vi "test.vi"() -> ()   [LabVIEW 2014]
panel:
  out "GetDisPlayData":i32(ring) items=["Success", "TimeOut", "CRCError", "WriteOutRange", "DeviceNotOpen", "ExceptionError"]
  out "arrayfloat":sgl[](array[numeric])
  in  "modeCode":i32(ring)=3 items=["CCH"=0, "CCL"=1, "CVH"=2, "CVL"=3, "CR"=4, "CP"=5, "CCDH"=6, "CCDL"=7, "OCP"=8, "DISCHARGE"=9, "AUTO"=12, "SEQ"=13, "LED"=14]
  out "错误输出":errorcluster
  out "Close":bool
  out "Open":bool
  in  "簇":T1
  in  "错误输入（无错误）":errorcluster
  # "-1861025792"
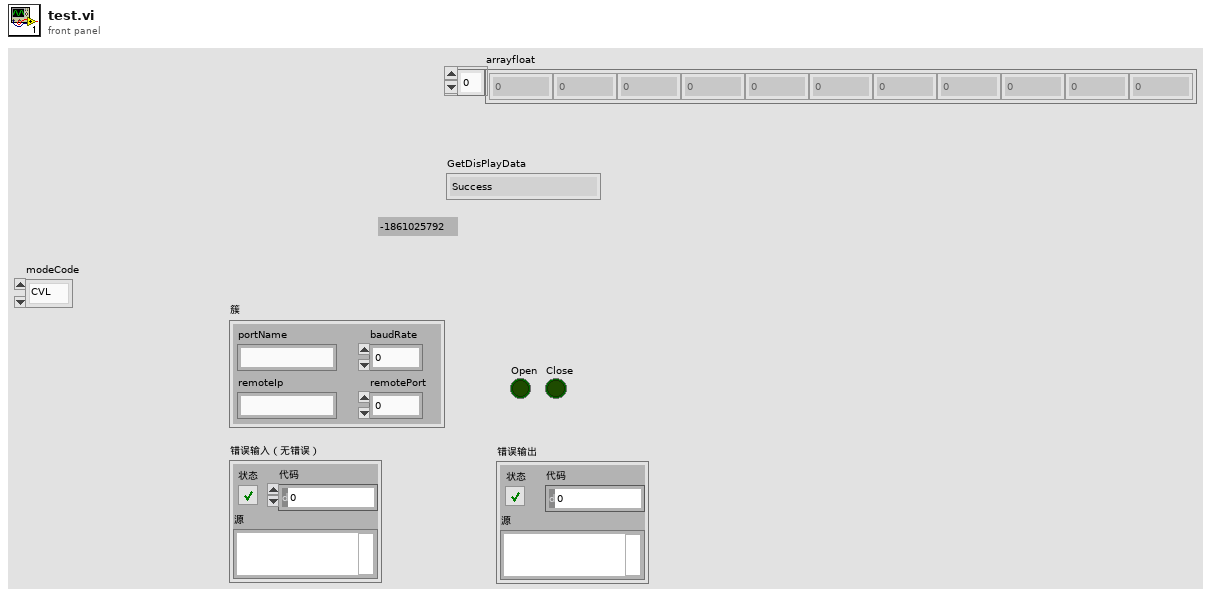
[diagram p1: front panel]
types:
  T1 = cluster{"portName":string, "baudRate":i32, "remoteIp":string, "remotePort":i32}
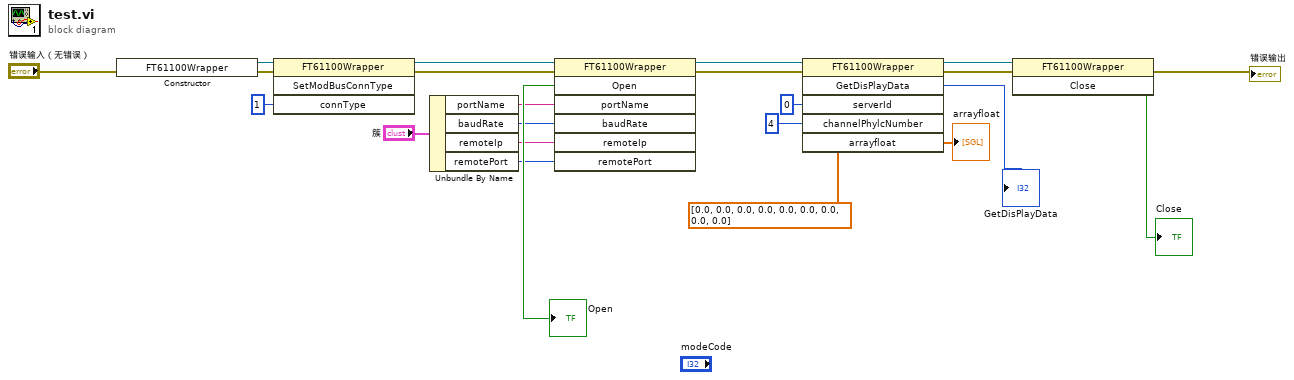
[diagram p0: block diagram]
diagram:
  n1 = constructor class="FT61100Wrapper"(error in="错误输入（无错误）") -> (reference out=w22:refnum<k24>, error out=w21:errorcluster)  [unwired: 2 in, 1 out]
  n2 = invoke class="FT61100Wrapper" method="SetModBusConnType"(reference=w22, error in=w21, "connType"=1) -> (reference out=w20:refnum<k24>, error out=w19:errorcluster)  [unwired: 1 in, 2 out]
  n3 = Unbundle By Name("簇") -> ("portName"=w13:string, "baudRate"=w12:i32, "remoteIp"=w11:string, "remotePort"=w10:i32)
  n4 = invoke class="FT61100Wrapper" method="Open"(reference=w20, error in=w19, "portName"=w13, "baudRate"=w12, "remoteIp"=w11, "remotePort"=w10) -> (reference out=w7:refnum<k24>, error out=w6:errorcluster, "Open"=→"Open":bool)  [unwired: 1 in, 4 out]
  n5 = invoke class="FT61100Wrapper" method="GetDisPlayData"(reference=w7, error in=w6, "serverId"=u8 0, "channelPhylcNumber"=4, "arrayfloat"=sgl[] [0.0, 0.0, 0.0, 0.0, 0.0, 0.0, 0.0, 0.0, 0.0]) -> (reference out=w9:refnum<k24>, error out=w8:errorcluster, "GetDisPlayData"=→"GetDisPlayData":i32, "arrayfloat"=→"arrayfloat":sgl[])  [unwired: 1 in, 2 out]
  n6 = invoke class="FT61100Wrapper" method="Close"(reference=w9, error in=w8) -> (error out=→"错误输出":errorcluster, "Close"=→"Close":bool)  [unwired: 1 in, 1 out]
